vi "GetCommonMessageData.vi"(8 "error in (no error)":errorcluster, 11 "MessageArgs":refnum<k24>) -> (0 "error out":errorcluster, 1 "State":string, 2 "Message":T1)   [LabVIEW 2017]
uses:
  <vilib>/addons/InsightCM/MessageBus/Base/controls/Message.ctl
  <vilib>/addons/InsightCM/MessageBus/Base/controls/MessageHeader.ctl
  <vilib>/addons/InsightCM/MessageBus/Base/controls/KeyValuePair.ctl
  C:/Program Files (x86)/National Instruments/LabVIEW 2017/vi.lib/addons/InsightCM/Binaries/LabviewMessageAdapter.dll
  Binaries/LabviewMessageAdapter.dll
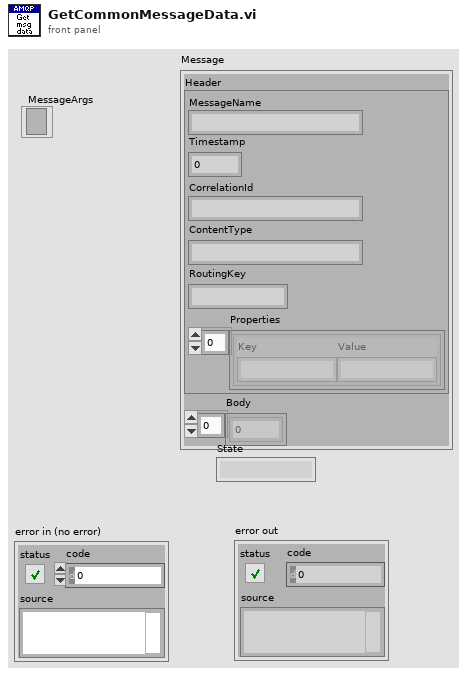
[diagram p1: front panel]
types:
  T1 = typedef "Message.ctl" = cluster{"Header":T2, "Body":u8[]}
  T2 = typedef "MessageHeader.ctl" = cluster{"MessageName":string, "Timestamp":i64, "CorrelationId":string, "ContentType":string, "RoutingKey":string, "Properties":T3[]}
  T3 = typedef "KeyValuePair.ctl" = cluster{"Key":string, "Value":string}
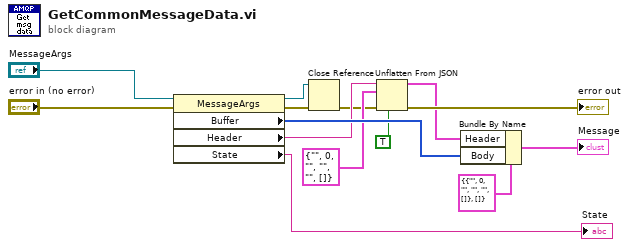
[diagram p0: block diagram]
diagram:
  n1 = property class="MessageArgs"(reference="MessageArgs", error in="error in (no error)") -> (reference out=w13:refnum<k24>, error out=w12:errorcluster, "Buffer"=w8:u8[], "Header"=w6:string, "State"=→"State":string)
  n2 = Close Reference(reference=w13, error in (no error)=w12) -> (error out=w5:errorcluster)
  n3 = Unflatten From JSON(JSON string=w6, type and defaults=T2 {"MessageName"="", "Timestamp"=0, "CorrelationId"="", "ContentType"="", "RoutingKey"="", "Properties"=[]} ("Header"), default null elements? (F)=TRUE, error in (no error)=w5) -> (value=w3:T2, error out=→"error out":errorcluster)  [unwired: 3 in]
  n4 = Bundle By Name(cluster=T1 {"Header"={"MessageName"="", "Timestamp"=0, "CorrelationId"="", "ContentType"="", "RoutingKey"="", "Properties"=[]}, "Body"=[]} ("Common"), "Header"=w3, "Body"=w8) -> (→"Message":T1)
